vi "Main.vi"() -> ()   [LabVIEW 2015]
doc: "The myRIO Project template acquires acceleration data from the onboard accelerometer and displays the changes of acceleration values in a waveform chart."
uses:
  <vilib>/NIOSC/Create Int32 Argument.vi
  <vilib>/myRIO/Common/Instrument Driver Framework/myRIO v1.0/UART/vis/myRIO v1.0 Close UART.vi
  <vilib>/NIOSC/Create Message_Single Arg.vi
  <vilib>/myRIO/Common/Instrument Driver Framework/Utilities/vis/FPGA Ref Manager.vi
  <vilib>/myRIO/Common/Instrument Driver Framework/myRIO v1.0/myRIO v1.0 Reset FPGA.vi
  <vilib>/myRIO/Common/Instrument Driver Framework/myRIO v1.0/IRQ/vis/myRIO v1.0 IRQ Info FGV.vi
  <vilib>/myRIO/Common/Instrument Driver Framework/myRIO v1.0/IRQ/vis/myRIO v1.0 Timer IRQ Info FGV.vi
  <vilib>/myRIO/Common/Instrument Driver Framework/myRIO v1.0/IRQ/vis/myRIO v1.0 ISR Agent.vi
  <vilib>/myRIO/Instrument Drivers/Utilities/Utilities.lvlib
  <vilib>/NIOSC/NI_OSC.lvlib
panel:
  out "error out":errorcluster
  in  "Stop":bool
  # "Overview: The myRIO Project template acquires acceleration data from the onboard accelerometer and displays the changes of acceleration values in a waveform chart.\nInstructions:\n1. Check the myRIO target IP address in the project and make sure the target IP address is correct. \n2. Run this VI."
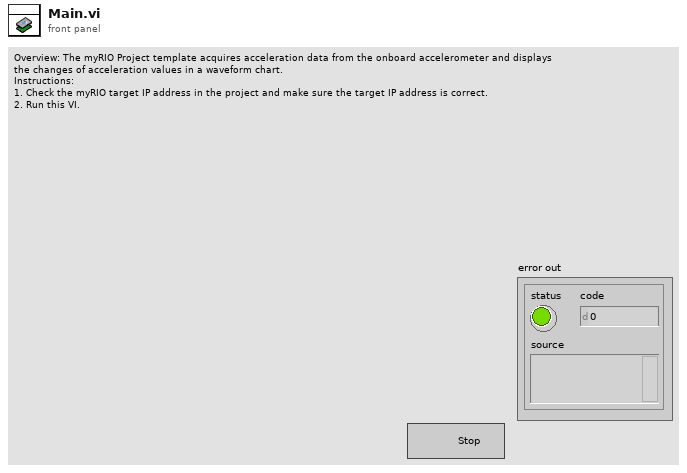
[diagram p1: front panel]
types:
  T1 = typedef "NI_OSC.lvlib/Argument.ctl" = cluster{"argument":string, "type tag":string}
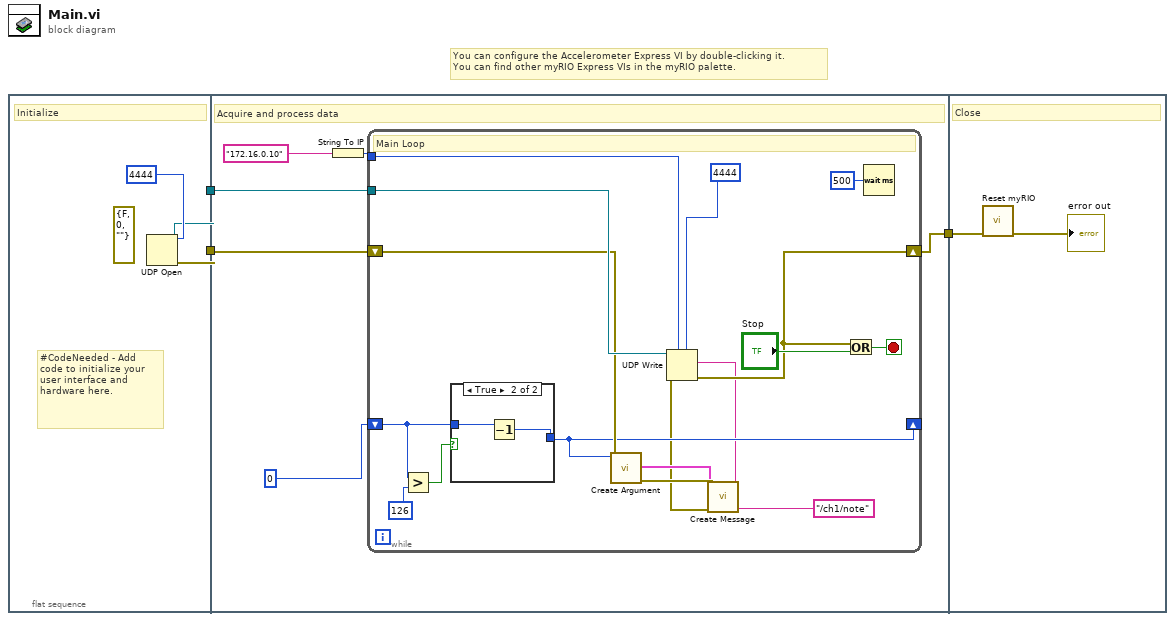
[diagram p0: block diagram]
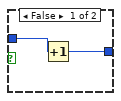
[diagram p2: hidden frame]
diagram:
  # "You can configure the Accelerometer Express VI by double-clicking it.\nYou can find other myRIO Express VIs in the myRIO palette."
  n1 = flat-sequence {
    tunnel: [w4] -> w3
    tunnel: [w5] -> w1
    tunnel: w3 -> [w12]
    tunnel: [w11] -> w2
    tunnel: w1 -> [w10]
    tunnel: w2 -> [w35]
    frame #0 {
      (unwired) errorcluster {"status"=FALSE, "code"=0, "source"=""} ("error in (no error)")
      # "#CodeNeeded - Add code to initialize your user interface and hardware here."
      # "Initialize"
      n2 = UDP Open(11:u16 4444 ("port")) -> (port=w5:refnum<k16>, 0:w4:errorcluster)  [unwired: 4 in, 1 out]
    }
    frame #1 {
      # "Acquire and process data"
      n3 = String To IP(1:"172.16.0.10" ("data")) -> (0:w8:u32)
      n4 = while {
        shift-right: [w24] -> w11
        shift-left: w12 -> [w21]
        tunnel: w10 -> [w26]
        tunnel: w8 -> [w23]
        shift-right: [w16] -> _
        shift-left: 0 -> [w18]
        stop <- w28 stop-if-true
        # "Main Loop"
        n5 = Greater?(x=w18, y=126) -> (0:w19:bool)
        n6 = case shown="True" w19 {
          tunnel: w18 -> [w31 w33]
          tunnel: [w30 w32] -> w16
          frame False {
            n7 = Increment(x=w31) -> (x+1=w30:i32)
          }
          frame True {
            n8 = Decrement(x=w33) -> (x-1=w32:i32)
          }
        }
        n9 = call-poly <vilib>:"Create Argument.vi"("error in"=w21, "int32 data"=w16) -> ("error out"=w20:errorcluster, "int32 argument"=w15:T1)  [unwired: 8 in]
        n10 = call-poly <vilib>:"Create Message.vi"("error in"=w20, "argument"=w15, "address pattern"="/ch1/note") -> ("error out"=w14:errorcluster, "message"=w13:string)  [unwired: 7 in]
        n11 = UDP Write(address=w23, port or service name=u16 4444 ("port"), connection ID=w26, data in=w13, 8:w14) -> (error out=w24:errorcluster)  [unwired: 1 in, 1 out]
        n12 = Or(x=w24, y="Stop") -> (x .or. y?=w28:bool)
        n13 = Wait (ms)(milliseconds to wait=u32 500) -> ()  [unwired: 1 out]
      }
    }
    frame #2 {
      # "Close"
      n14 = call <vilib>:"Reset myRIO.vi"("error in (no error)"=w35) -> ("error out"=→"error out":errorcluster)  [unwired: 10 in]
    }
  }
